vi "Lezeti_Power_Monitor_24_d.vi"() -> ()   [LabVIEW 2014]
uses:
  <vilib>/addons/Electrical Power/Basic/Controls/Vector Diagram/EPX Vector Diagram.xctl
  <vilib>/measure/madcrms.llb/Basic Averaged DC-RMS for N Chan.vi
  <vilib>/measure/madcrms.llb/Basic Averaged DC-RMS for 1 Chan.vi
  <vilib>/addons/Electrical Power/Basic/Measurement/Fundamental Vector (N Channels).vi
  <vilib>/addons/Electrical Power/Basic/Measurement/Power (1 Channel).vi
  <vilib>/Utility/file.llb/Write To Spreadsheet File (DBL).vi
  <vilib>/measure/NI_MAPro.lvlib
  <vilib>/addons/Electrical Power/Basic/NI_EP_Basic.lvlib
panel:
  out "Current Vector":cdb[](array[numeric])
  out "Current Vector Diagram":cdb[](xcontrol)
  out "voltage vector":cdb[](array[numeric])
  out "Voltage Vector Diagram":cdb[](xcontrol)
  out "Reactive Power (VAR) EPS Check 2":dbl
  out "Power Factor EPS Check":dbl
  out "Apparent Power (VA) EPS Check":dbl
  out "Average Power (Watts) EPS Check":dbl
  in  "High Resolution Waveform Data Path":path
  out "Power Factor":dbl
  in  "Average Power Output File":path
  out "Run Date":string
  out "Run Time":string
  out "Elapsed Time (s)":dbl
  out "Apparent Power (VA)":dbl
  out "Average Power (Watts)":dbl
  out "Instantaneous Power Waveform":waveform(dbl)[](graph)
  out "RMS Voltage L1-L2":dbl
  out "L2 RMS Current":dbl
  out "L1 RMS Current":dbl
  in  "Burden Resistor (ohms) (1000)":dbl
  in  "CT Ratio (Iout/Iin) (.0003332)":dbl
  in  "Acquire Sample Size (1000)":dbl
  in  "Acquire Rate (Hz) (1000)":dbl
  in  "Acquire Timeout (1000)":dbl
  out "Line 2 Current Waveform":waveform(dbl)[](graph)
  out "Line 1 Current Waveform":waveform(dbl)[](graph)
  out "Voltage L1-L2":waveform(dbl)[](graph)
  in  "stop":bool
  # "For Lezeti Air Conditioning System (Greenpath Tech)\nBy Matsu Thornton\nJuly 2016"
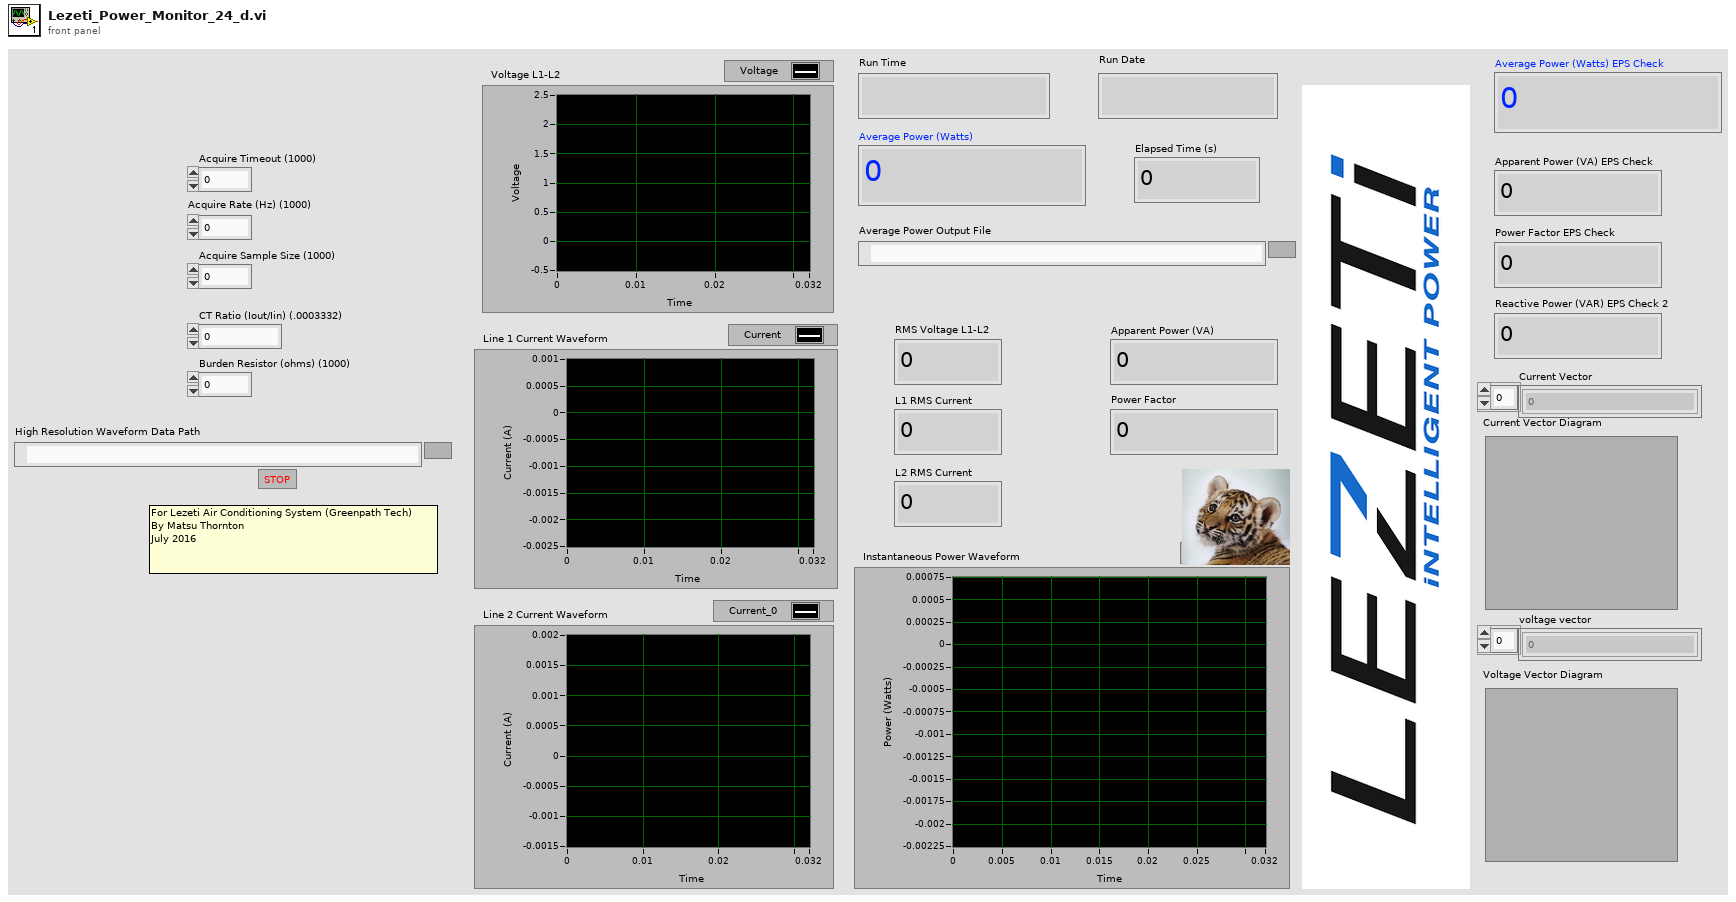
[diagram p1: front panel]
types:
  T1 = typedef "NI_EP_Basic.lvlib/basic_Power Value.ctl" = cluster{"active power [W]":dbl, "apparent power [VA]":dbl, "reactive power [VAR]":dbl, "power factor":dbl}
  T2 = typedef "NI_Matrix.lvlib/RealMatrix.ctl" = dbl[][]
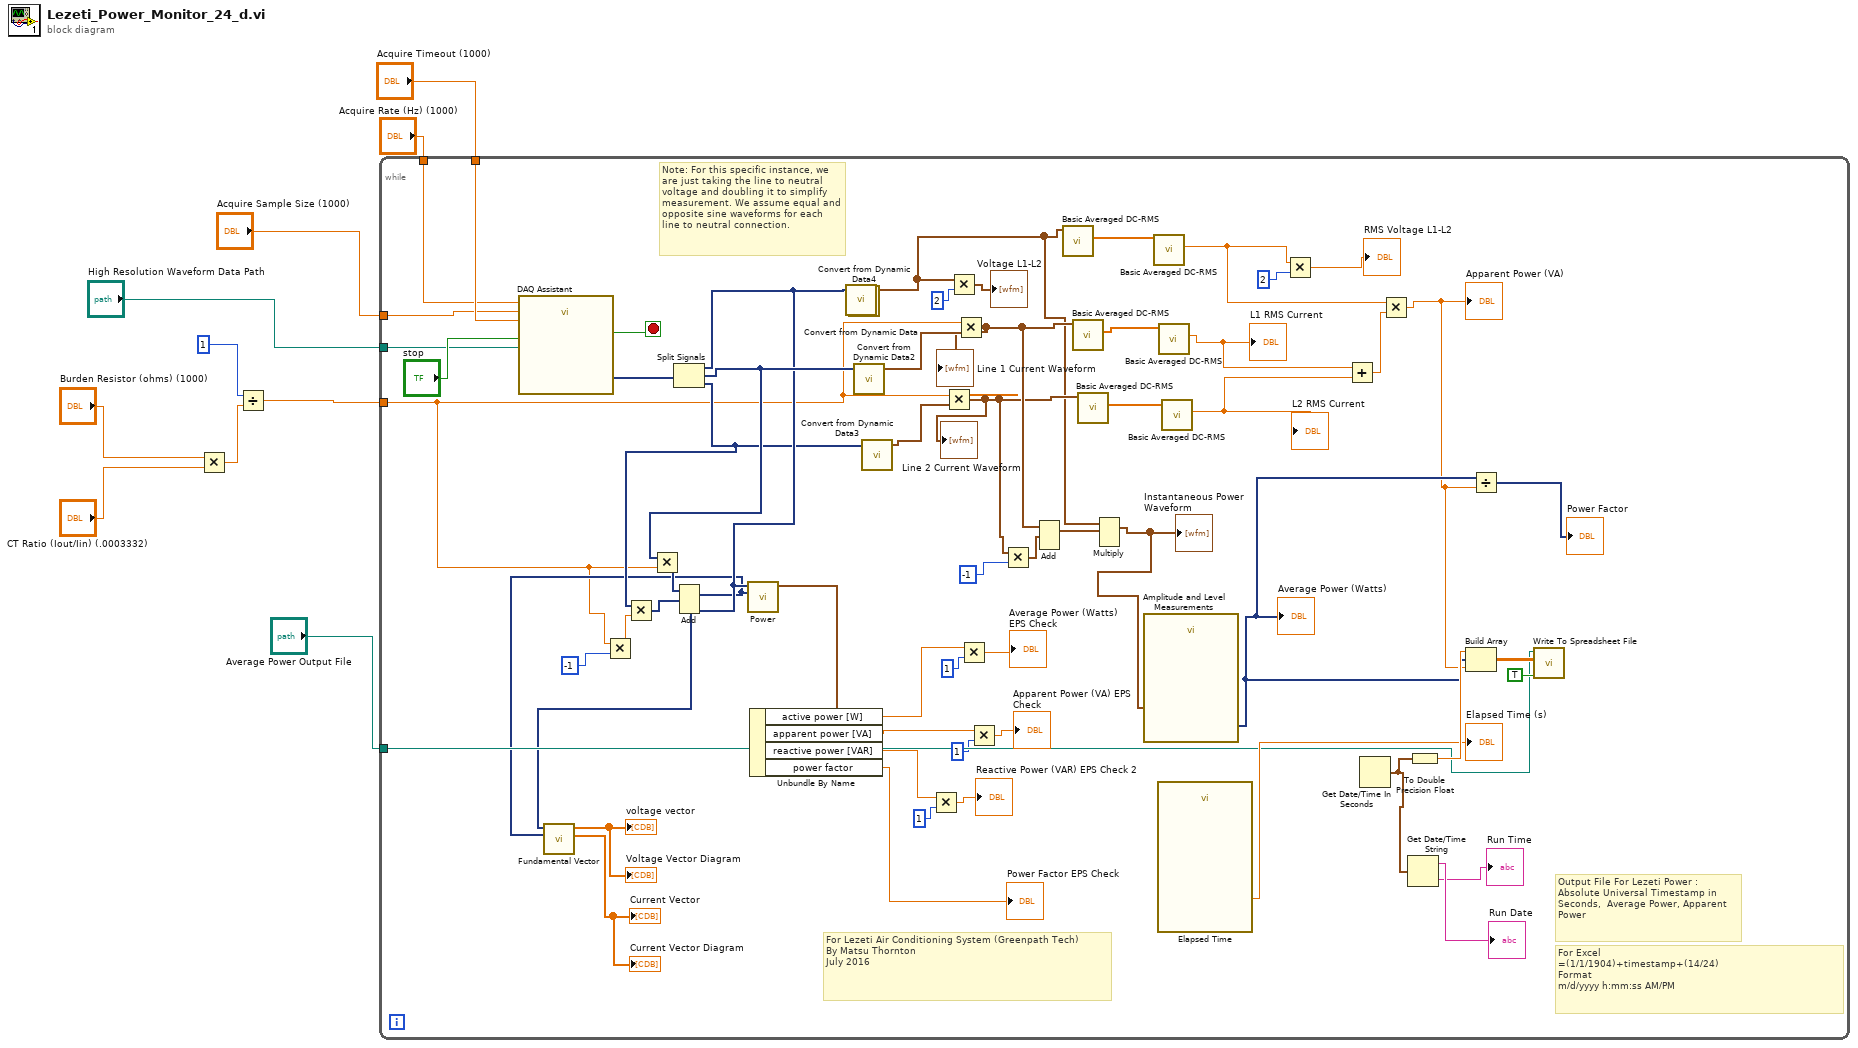
[diagram p0: block diagram]
diagram:
  n1 = Multiply(x="Burden Resistor (ohms) (1000)", y="CT Ratio (Iout/Iin) (.0003332)") -> (x*y=w4:dbl)
  n2 = Divide(x=1, y=w4) -> (x/y=w3:dbl)
  n3 = while {
    tunnel: "Acquire Timeout (1000)" -> [w70]
    tunnel: "Acquire Rate (Hz) (1000)" -> [w47]
    tunnel: "Acquire Sample Size (1000)" -> [w46]
    tunnel: w3 -> [w12]
    tunnel: "Average Power Output File" -> [w50]
    tunnel: "High Resolution Waveform Data Path" -> [w45]
    stop <- w44 stop-if-true
    # "Note: For this specific instance, we are just taking the line to neutral voltage and doubling it to simplify measurement. We assume equal and opposite sine waveforms for each line to neutral connection."
    # "For Excel\n=(1/1/1904)+timestamp+(14/24)\nFormat\nm/d/yyyy h:mm:ss AM/PM"
    # "Output File For Lezeti Power :\nAbsolute Universal Timestamp in Seconds,  Average Power, Apparent Power"
    # "For Lezeti Air Conditioning System (Greenpath Tech)\nBy Matsu Thornton\nJuly 2016"
    n4 = call "DAQ Assistant"("rate"=w47, "number of samples"=w46, "timeout (s)"=w70, "stop (F)"="stop", "file path"=w45) -> ("data"=w33:dynamicdata, "stopped"=w44:bool)  [unwired: 11 in, 2 out]
    n5 = Multiply(x=w12, y=-1) -> (x*y=w11:dbl)
    n6 = Split Signals(w33) -> (w20:dynamicdata, w28:dynamicdata, w17:dynamicdata)  [unwired: 3 in]
    n7 = Multiply(x=w17, y=w11) -> (x*y=w15:dynamicdata)
    n8 = Multiply(x=w28, y=w12) -> (x*y=w16:dynamicdata)
    n9 = Add(1:w15, 2:w16) -> (0:w14:dynamicdata)  [unwired: 1 in, 1 out]
    n10 = call-poly <vilib>:"Fundamental Vector.vi"("current waveforms"=w14, "voltage waveforms"=w20) -> ("current fundamental vectors"=→"Current Vector Diagram" →"Current Vector":cdb[], "voltage fundamental vectors"=→"Voltage Vector Diagram" →"voltage vector":cdb[])  [unwired: 6 in, 2 out]
    n11 = call-poly <vilib>:"Power.vi"("current waveform"=w14, "voltage waveform"=w20) -> ("power value"=w32:T1)  [unwired: 8 in, 1 out]
    n12 = Unbundle By Name(w32) -> ("active power [W]"=w30:dbl, "apparent power [VA]"=w25:dbl, "reactive power [VAR]"=w21:dbl, "power factor"=→"Power Factor EPS Check":dbl)
    n13 = call "Convert from Dynamic Data"("Dynamic Data Type"=w20) -> ("Array of Waveform"=w35:waveform(dbl)[])  [unwired: 3 in]
    n14 = call "Convert from Dynamic Data4"() -> ()  [unwired: 4 in, 1 out]
    n15 = call "Convert from Dynamic Data2"("Dynamic Data Type"=w28) -> ("Array of Waveform"=w65:waveform(dbl)[])  [unwired: 3 in]
    n16 = call "Convert from Dynamic Data3"("Dynamic Data Type"=w17) -> ("Array of Waveform"=w64:waveform(dbl)[])  [unwired: 3 in]
    n17 = Multiply(x=w21, y=1) -> (x*y=→"Reactive Power (VAR) EPS Check 2":dbl)
    n18 = Multiply(x=w12, y=w64) -> (x*y=w42:waveform(dbl)[])
    "Line 2 Current Waveform" <- w42
    n19 = Multiply(x=w35, y=2) -> (x*y=→"Voltage L1-L2":waveform(dbl)[])
    n20 = Multiply(x=w12, y=w65) -> (x*y=w61:waveform(dbl)[])
    "Line 1 Current Waveform" <- w61
    n21 = Multiply(x=w30, y=1) -> (x*y=→"Average Power (Watts) EPS Check":dbl)
    n22 = Multiply(x=w25, y=1) -> (x*y=→"Apparent Power (VA) EPS Check":dbl)
    n23 = Multiply(x=w42, y=-1) -> (x*y=w43:waveform(dbl)[])
    n24 = Add(1:w43, 2:w61) -> (0:w63:waveform(dbl)[])  [unwired: 1 in, 1 out]
    n25 = call-poly <vilib>:"Basic Averaged DC-RMS.vi"("signals in"=w35) -> ("RMS values"=w68:dbl[])  [unwired: 7 in, 3 out]
    n26 = call-poly <vilib>:"Basic Averaged DC-RMS.vi"("signals in"=w61) -> ("RMS values"=w67:dbl[])  [unwired: 7 in, 3 out]
    n27 = call-poly <vilib>:"Basic Averaged DC-RMS.vi"("signals in"=w42) -> ("RMS values"=w66:dbl[])  [unwired: 7 in, 3 out]
    n28 = Multiply(1:w63, 2:w35) -> (0:w62:waveform(dbl)[])  [unwired: 1 in, 1 out]
    "Instantaneous Power Waveform" <- w62
    n29 = call "Amplitude and Level Measurements"("Signals"=w62) -> ("Mean (DC)"=w49:dynamicdata)  [unwired: 13 in, 1 out]
    "Average Power (Watts)" <- w49
    n30 = call-poly <vilib>:"Basic Averaged DC-RMS.vi"("signal in"=w68) -> ("RMS value"=w38:dbl)  [unwired: 7 in, 3 out]
    n31 = call "Elapsed Time"() -> ("Elapsed Time (s)"=→"Elapsed Time (s)":dbl)  [unwired: 12 in, 7 out]
    n32 = call-poly <vilib>:"Basic Averaged DC-RMS.vi"("signal in"=w67) -> ("RMS value"=w60:dbl)  [unwired: 7 in, 3 out]
    "L1 RMS Current" <- w60
    n33 = call-poly <vilib>:"Basic Averaged DC-RMS.vi"("signal in"=w66) -> ("RMS value"=w59:dbl)  [unwired: 7 in, 3 out]
    "L2 RMS Current" <- w59
    n34 = Multiply(x=w38, y=2) -> (x*y=→"RMS Voltage L1-L2":dbl)
    n35 = Add(x=w60, y=w59) -> (x+y=w58:dbl)
    n36 = Get Date/Time In Seconds() -> (seconds since 1Jan1904=w54:timestamp)
    n37 = Multiply(x=w38, y=w58) -> (x*y=w40:dbl)
    "Apparent Power (VA)" <- w40
    n38 = Get Date/Time String(seconds (now)=w54) -> (date string=→"Run Date":string, time string=→"Run Time":string)  [unwired: 2 in]
    n39 = To Double Precision Float(number=w54) -> (double precision float=w55:dbl)
    n40 = Build Array(w55, w49, w40) -> (w56:T2)
    n41 = Divide(x=w49, y=w40) -> (x/y=→"Power Factor":dynamicdata)
    n42 = call-poly <vilib>:"Write To Spreadsheet File.vi"("append to file? (new file:F)"=TRUE, "2D data"=w56, "file path (dialog if empty)"=w50) -> ()  [unwired: 5 in, 1 out]
  }
